vi "FTW-HTTPClient-POST-Multipart.vi"(0 "HTTP Client":refnum<class "FTW-HTTPClient.lvclass">, 5 "Endpoint":string, 7 "Multipart Values":T1[](array[typedef]), 11 "error in":errorcluster) -> (4 "HTTP Client out":refnum<class "FTW-HTTPClient.lvclass">, 6 "Response Headers":string, 8 "Response Body":string, 15 "error out":errorcluster)   [LabVIEW 2012, in "FTW-HTTPClient.lvclass"]
uses:
  FTW-HTTPClient.lvclass
  FTW-HTTPClient-MultipartData.ctl
  Utils/FTW-Web-MIMEtype.ctl
  FTW-HTTPClient.lvclass/FTW-HTTPClient.ctl
panel:
  # "Inputs"
  # "Outputs"
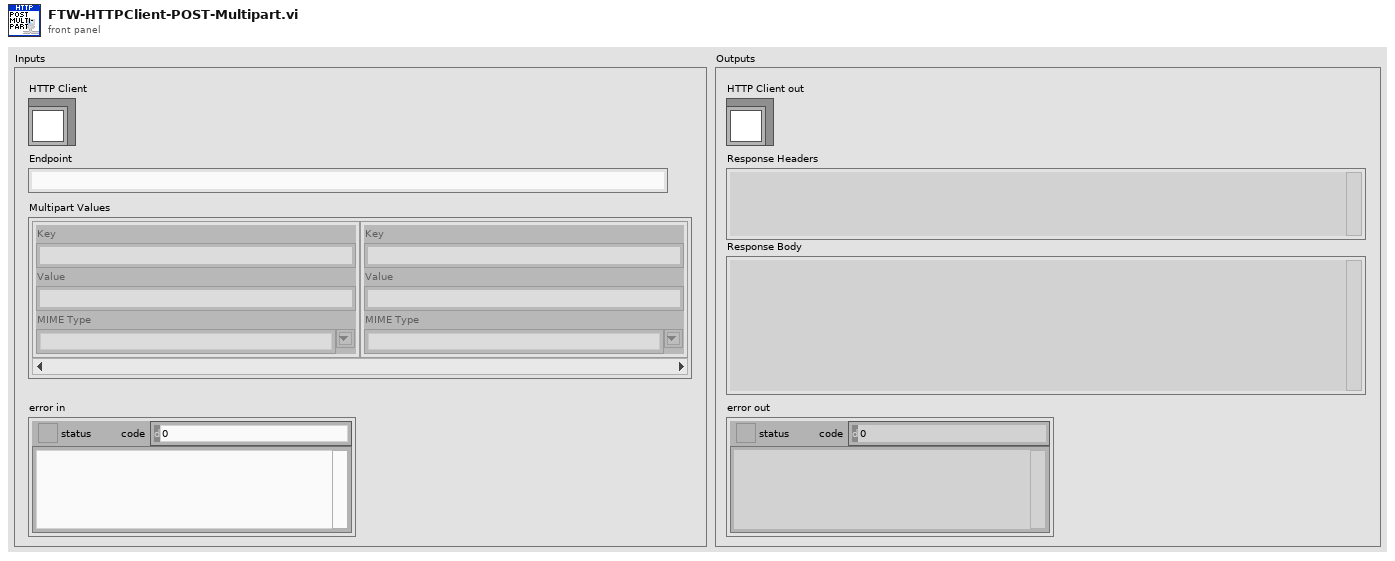
[diagram p1: front panel]
types:
  T1 = typedef "FTW-HTTPClient.lvclass/FTW-HTTPClient-MultipartData.ctl" = cluster{"Key":string, "Value":string, "MIME Type":T2}
  T2 = typedef "FTW-Web-MIMEtype.ctl" = string
  T3 = cluster{"Name":string, "Value":string, "File":path, "Filename":string, "MIME type":string}
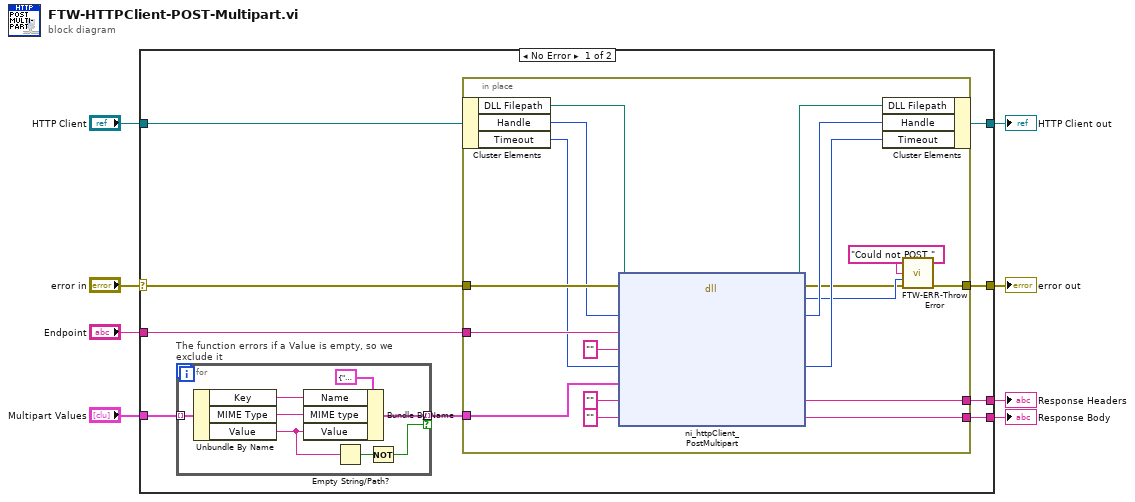
[diagram p0: block diagram]
diagram:
  n1 = case shown="No Error" "error in" {
    selector: "error in" -> [w16 w45]
    tunnel: "Endpoint" -> [w14 _]
    tunnel: [w13 w45] -> w7
    tunnel: "HTTP Client" -> [w17 w44]
    tunnel: [w15 w44] -> w6
    tunnel: [w12 _] -> w3
    tunnel: [w11 _] -> w2
    tunnel: "Multipart Values" -> [w9 _]
    frame No Error {
      n2 = for "The function errors if a Value is empty, so we exclude it" {
        tunnel: [w25] -> w10 mode=indexing if=w19
        tunnel: w9 -> [w24] mode=indexing
        n3 = Unbundle By Name(w24) -> ("Key"=w23:string, "MIME Type"=w22:T2, "Value"=w18:string)
        n4 = Bundle By Name(cluster=T3 {"Name"="", "Value"="", "File"=path "", "Filename"="", "MIME type"="application/octet-stream"} ("Element"), "Name"=w23, "MIME type"=w22, "Value"=w18) -> (w25:T3)
        n5 = Empty String/Path?(string/path=w18) -> (empty?=w20:bool)
        n6 = Not(x=w20) -> (.not. x?=w19:bool)
      }
      n7 = in-place {
        in-place-border: w16 -> [w41]
        in-place-border: w14 -> [w39]
        in-place-border: w10 -> [w36]
        in-place-border: [w42] -> w13
        in-place-border: [w27] -> w12
        in-place-border: [w26] -> w11
        n8 = in-place-cluster #1(w17) -> ("DLL Filepath"=w31:path, "Handle"=w40:u32, "Timeout"=w37:i32)
        n9 = dll-call lib="ni_httpClient.*" fn="ni_httpClient_PostMultipart"(path in=w31, error in=w41, "Handle"=w40, "Endpoint"=w39, "Output Filepath"="", "Timeout"=w37, "Multipart Data"=w36, "Response Header"="", "Response Body"="") -> (path out=w30:path, error out=w28:errorcluster, "Return"=w29:i32, "Handle"=w33:u32, "Timeout"=w32:i32, "Response Header"=w27:string, "Response Body"=w26:string)  [unwired: 4 in]
        n10 = in-place-cluster #1("DLL Filepath"=w30, "Handle"=w33, "Timeout"=w32) -> (w15:refnum<class "FTW-HTTPClient.lvclass">)
        n11 = call "FTW-ERR-ThrowError.vi"("Error Message"="Could not POST.", "Error Code"=w29, "error in"=w28) -> ("error out"=w42:errorcluster)  [unwired: 12 in]
      }
    }
    frame Error {
    }
  }
  "error out" <- w7
  "HTTP Client out" <- w6
  "Response Headers" <- w3
  "Response Body" <- w2
